vi "process.vi"(8 "error in":errorcluster, 10 "responder in":refnum<class "https responder.lvclass">, 11 "Basic HTTP server in":refnum<class "Basic HTTPS server.lvclass">) -> (0 "error out":errorcluster, 2 "responder out":refnum<class "https responder.lvclass">, 3 "Basic HTTP server out":refnum<class "Basic HTTPS server.lvclass">)   [LabVIEW 2016, in "Basic HTTPS server.lvclass"]
uses:
  Basic HTTPS server.lvclass
  HTTP responder/https responder.lvclass
  Basic HTTPS server.lvclass/Basic HTTPS server.ctl
  HTTP handler dataset/HTTPS handler dataset.lvclass
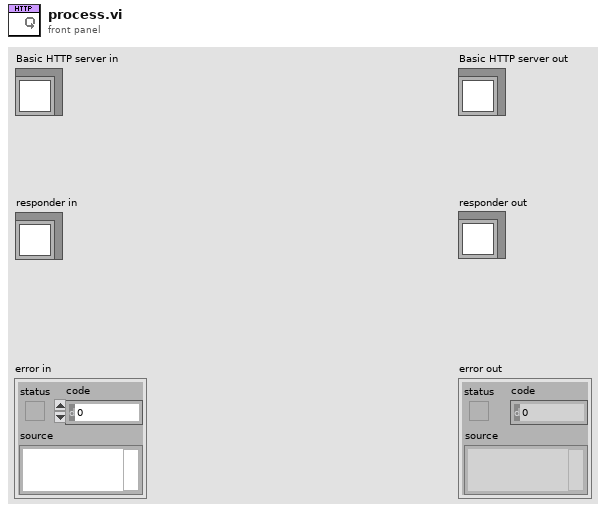
[diagram p1: front panel]
types:
  T1 = typedef "Basic HTTPS server.lvclass/http handler ref.ctl" = refnum<vi>
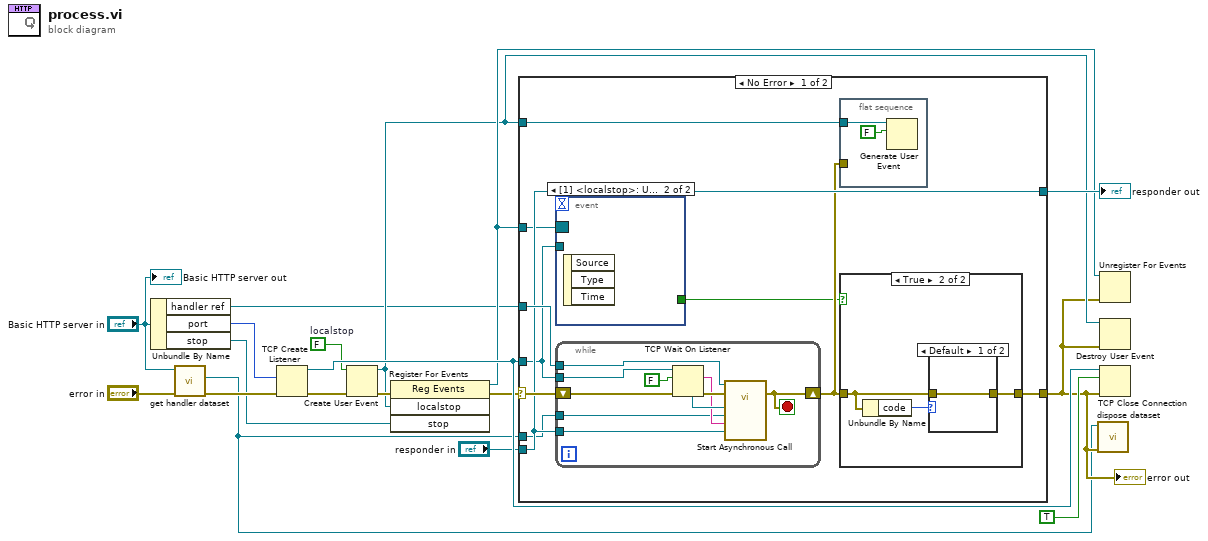
[diagram p0: block diagram]
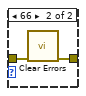
[diagram p3: hidden frame]
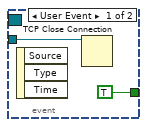
[diagram p4: hidden frame]
diagram:
  w10 = FALSE  # localstop
  n1 = Unbundle By Name("Basic HTTP server in") -> ("handler ref"=w3:T1, "port"=w4:u16, "stop"=w5:refnum<user-event>)
  n2 = call "get handler dataset.vi"("error in"="error in", "Basic HTTP server in"="Basic HTTP server in") -> ("error out"=w6:errorcluster, "basic HTTP handler dataset"=w1:refnum<class "HTTPS handler dataset.lvclass">)  [unwired: 8 in]
  n3 = TCP Create Listener(8:w6, 10:w4) -> (0:w15:errorcluster, 3:w18:refnum<k5>)  [unwired: 3 in, 1 out]
  n4 = Create User Event(user event datatype=w10, error in=w15) -> (user event=w9:refnum<user-event>, error out=w11:errorcluster)
  n5 = register-events(error in=w11, w9, w5) -> (reference out=w12:refnum<event-registration>, error out=w13:errorcluster)  [unwired: 1 in]
  n6 = case shown="No Error" w13 {
    selector: w13 -> [w28 w51]
    tunnel: [w21 w51] -> w2
    tunnel: w18 -> [w25 _]
    tunnel: w3 -> [w27 _]
    tunnel: "responder in" -> [w26 w50]
    tunnel: [w26 w50] -> w14
    tunnel: w12 -> [w24 _]
    tunnel: w9 -> [w23 _]
    tunnel: w1 -> [w19 _]
    frame No Error {
      n7 = event shown="[1] <localstop>: User Event" {
        selector: w24 -> [_ _]
        dyn-events: _ -> [_ _]
        timeout: _ -> [_ _]
        tunnel: w25 -> [w39 _]
        tunnel: [TRUE _] -> w20
        event User Event {
          n8 = event-data() -> ()  [unwired: 1 in, 3 out]
          n9 = TCP Close Connection(connection ID=w39) -> ()  [unwired: 2 in, 2 out]
        }
        event User Event {
          n10 = event-data() -> ()  [unwired: 1 in, 3 out]
        }
      }
      n11 = while {
        shift-right: [w46] -> w22
        shift-left: w28 -> [w49]
        tunnel: w25 -> [w48]
        tunnel: w27 -> [w45]
        tunnel: w26 -> [w43]
        tunnel: w19 -> [w40]
        stop <- w46 stop-if-true
        n12 = TCP Wait On Listener(8:w49, 10:FALSE ("resolve remote address (T)"), 11:w48) -> (0:w47:errorcluster, 2:w41:string, 4:w44:refnum<k5>)  [unwired: 1 in, 2 out]
        n13 = call-by-ref "Start Asynchronous Call"(reference=w45, error in=w47, "http responder"=w43, "remote address"=w41, "basic HTTP handler dataset"=w40, "connection"=w44) -> (error out=w46:errorcluster)  [unwired: 8 in, 1 out]
      }
      n14 = flat-sequence {
        tunnel: w22 -> [_]
        tunnel: w23 -> [w37]
        frame #0 {
          n15 = Generate User Event(user event=w37, event data cluster=FALSE ("event data")) -> ()  [unwired: 2 in, 2 out]
        }
      }
      n16 = case shown="True" w20 {
        tunnel: w22 -> [w29 w31]
        tunnel: [w29 w32] -> w21
        frame False {
        }
        frame True {
          n17 = Unbundle By Name(w31) -> ("code"=w30:i32)
          n18 = case shown="Default" w30 {
            tunnel: w31 -> [w33 w35]
            tunnel: [w33 w34] -> w32
            frame Default {
            }
            frame 66 {
              n19 = call <vilib>:"Clear Errors.vi"("error in (no error)"=w35) -> ("error out"=w34:errorcluster)  [unwired: 5 in, 1 out]
            }
          }
        }
      }
    }
    frame Error {
    }
  }
  "error out" <- w2
  "responder out" <- w14
  n20 = call "dispose dataset.vi"("error in"=w2, "basic HTTP handler dataset in"=w1) -> ()  [unwired: 9 in, 1 out]
  n21 = Unregister For Events(event registration refnum=w12, error in=w2) -> ()  [unwired: 1 out]
  n22 = Destroy User Event(user event=w9, error in=w2) -> ()  [unwired: 1 out]
  n23 = TCP Close Connection(connection ID=w18, abort (F)=TRUE, error in (no error)=w2) -> ()  [unwired: 2 out]
  "Basic HTTP server out" <- "Basic HTTP server in"
